vi "Start Module.vi"(8 "error in (no error)":errorcluster, 9 "Marca":T1, 10 "Com Port":refnum<visa-resource-name>, 11 "Run as Singleton? (F)":bool) -> (0 "error out":errorcluster, 1 "Wait for Event Sync?":bool, 2 "Multiple_uC Broadcast Events":T2, 3 "Module ID":i32)   [LabVIEW 2019, in "Multiple_uC.lvlib"]
doc: "Launches the Module Main.vi.\n_____\nBased on Delacor QMH Project Template 5.0.0.82."
uses:
  Multiple_uC.lvlib
  Broadcast Events--cluster.ctl
  Did Init Argument--cluster.ctl
  Status Updated Argument--cluster.ctl
  Error Reported Argument--cluster.ctl
  Stop Argument--cluster.ctl
  Get Module Execution Status Argument--cluster.ctl
  Clase Padre/Marca.ctl
  Module Running State--enum.ctl
  <vilib>/Delacor/Delacor QMH/Libraries/Cloneable Module Admin_class/Delacor_lib_QMH_Cloneable Module Admin.lvclass
  C:/Program Files/National Instruments/LabVIEW 2019/vi.lib/Delacor/Delacor QMH/Libraries/Module Admin_class/Delacor_lib_QMH_Module Admin.lvclass
  VI Reference Management/Main VI Type--strict_vi_ref.ctl
  <vilib>/Delacor/Delacor QMH/Libraries/Cloneable Module Admin_class/Delacor_lib_QMH_Cloneable Module Admin.lvclass/Delacor_lib_QMH_Cloneable Module Admin.ctl
  <vilib>/Delacor/Delacor QMH/Libraries/Module Admin_class/Delacor_lib_QMH_Module Admin.lvclass/Delacor_lib_QMH_Module Admin.ctl
  <vilib>/Delacor/Delacor QMH/Libraries/Cloneable Module Admin_class/Delacor_lib_QMH_Set Module ID.vi
  <vilib>/Delacor/Delacor QMH/Libraries/Module Admin_class/Delacor_lib_QMH_Set External Launch.vi
  <vilib>/Utility/error.llb/Error Cluster From Error Code.vi
  <vilib>/ErrorRing/Error Ring.xnode
  Clone Registration/Clone Registration.lvlib
  VI Reference Management/VI Reference Management.lvlib
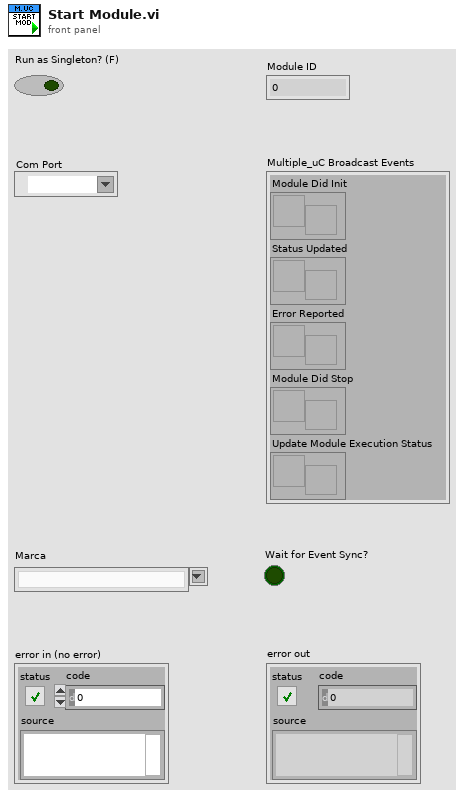
[diagram p1: front panel]
types:
  T1 = typedef "Marca.ctl" = string
  T2 = typedef "Multiple_uC.lvlib/Broadcast Events--cluster.ctl" = cluster{"Module Did Init":refnum<user-event>, "Status Updated":refnum<user-event>, "Error Reported":refnum<user-event>, "Module Did Stop":refnum<user-event>, "Update Module Execution Status":refnum<user-event>}
  T3 = typedef "Multiple_uC.lvlib/Module Running State--enum.ctl" = enum16{"Not Running", "Running as Cloneable", "Running as Singleton"}
  T4 = enum32{"Bad", "Idle", "Run top level", "Running"}
  T5 = typedef "Multiple_uC.lvlib/VI Reference Management.lvlib/Main VI Type--strict_vi_ref.ctl" = refnum<vi>
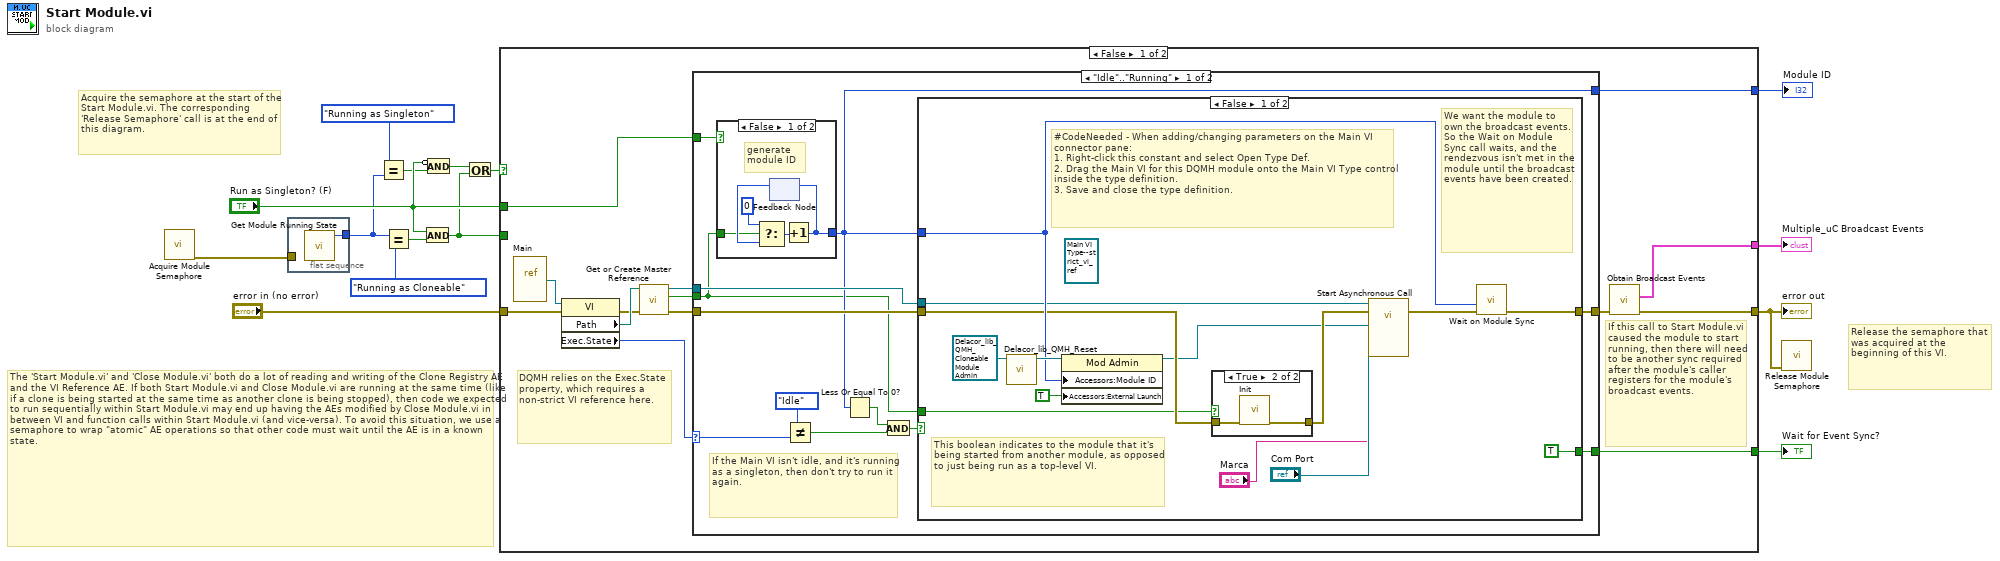
[diagram p0: block diagram]
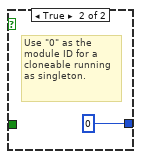
[diagram p2: hidden frame]
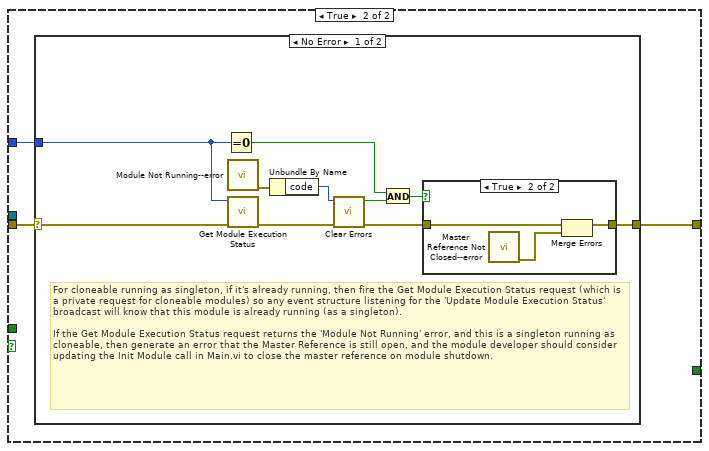
[diagram p4: hidden frame]
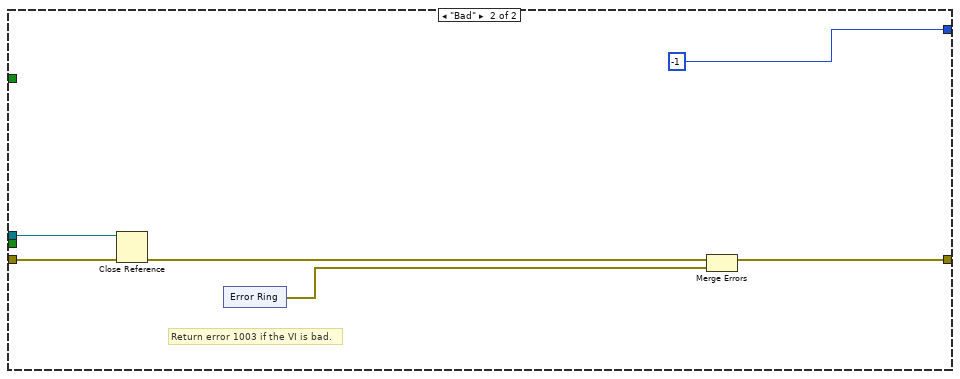
[diagram p7: hidden frame]
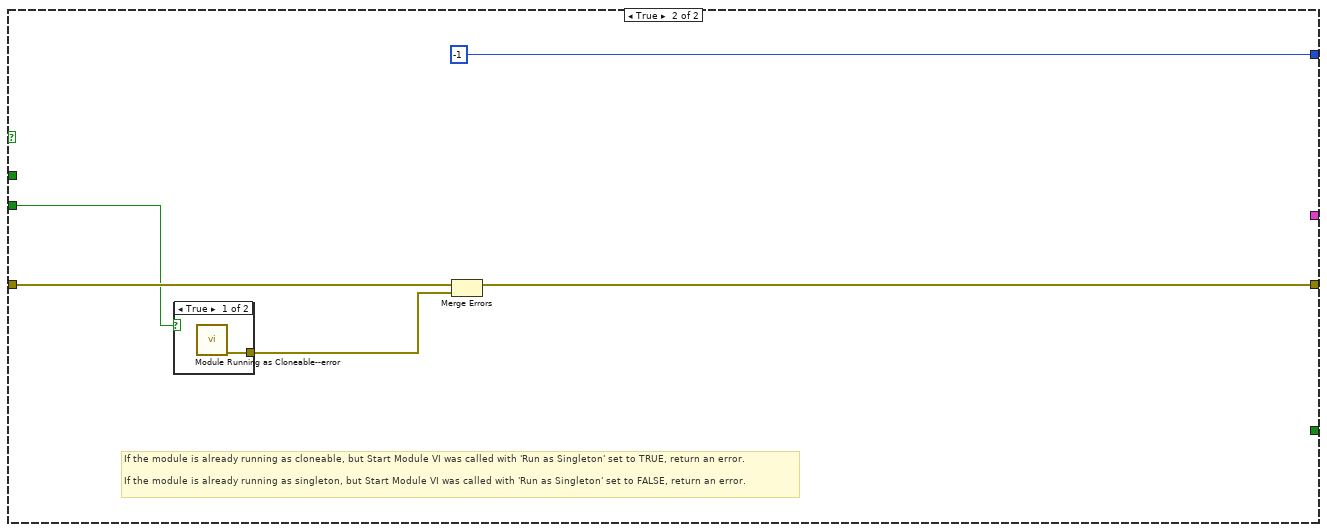
[diagram p8: hidden frame]
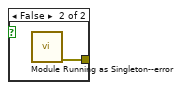
[diagram p9: hidden frame]
diagram:
  # "Release the semaphore that was acquired at the beginning of this VI."
  # "The 'Start Module.vi' and 'Close Module.vi' both do a lot of reading and writing of the Clone Registry AE and the VI Reference AE. If both Start Module.vi and Close Module.vi are running at the same time (like if a clone is being started at the same time as another clone is being stopped), then code we expected to run sequentially within Start Module.vi may end up having the AEs modified by Close Module.vi in between VI and function calls within Start Module.vi (and vice-versa). To avoid this situation, we use a semaphore to wrap \"atomic\" AE operations so that other code must wait until the AE is in a known state."
  # "Acquire the semaphore at the start of the Start Module.vi. The corresponding 'Release Semaphore' call is at the end of this diagram."
  n1 = call "Acquire Module Semaphore.vi"() -> ("error out"=w2:errorcluster)  [unwired: 11 in]
  n2 = flat-sequence {
    tunnel: [w16] -> w5
    tunnel: w2 -> [_]
    frame #0 {
      n3 = call "Get Module Running State.vi"() -> ("Module Running State"=w16:T3)  [unwired: 11 in]
    }
  }
  n4 = Equal?(x=Module_Running_State--enum."Running as Singleton", y=w5) -> (x = y?=w6:bool)
  n5 = Equal?(x=w5, y=Module_Running_State--enum."Running as Cloneable") -> (x = y?=w10:bool)
  n6 = And(x="Run as Singleton? (F)", y=w10) -> (x .and. y?=w3:bool)
  n7 = Compound Arithmetic op=AND(invert "Run as Singleton? (F)", w6) -> (w8:bool)
  n8 = Or(x=w8, y=w3) -> (x .or. y?=w9:bool)
  n9 = case shown="False" w9 {
    tunnel: "error in (no error)" -> [w30 w98]
    tunnel: [w28 w97] -> w1
    tunnel: [w27 _] -> w14
    tunnel: [w26 _] -> w13
    tunnel: [w22 -1] -> w12
    tunnel: "Run as Singleton? (F)" -> [w18 _]
    tunnel: w3 -> [_ w94]
    frame False {
      # "DQMH relies on the Exec.State property, which requires a non-strict VI reference here."
      # "If this call to Start Module.vi caused the module to start running, then there will need to be another sync required after the module's caller registers for the module's broadcast events."
      n10 = vi-ref "Main.vi"() -> (w21:refnum<vi>)
      n11 = property class="VI"(reference=w21, error in=w30) -> (error out=w24:errorcluster, "Path"=w25:path, "Exec.State"=w19:T4)  [unwired: 1 out]
      n12 = call "Get or Create Master Reference.vi"("error in (no error)"=w24, "Main VI Path"=w25) -> ("error out"=w23:errorcluster, "New Reference Created"=w17:bool, "Master Reference"=w20:T5)  [unwired: 7 in]
      n13 = case shown="\"Idle\"..\"Running\"" w19 {
        selector: w19 -> [w38 _]
        tunnel: w23 -> [w42 w89]
        tunnel: w20 -> [w40 w88]
        tunnel: [w39 w86] -> w29
        tunnel: [w41 _] -> w26
        tunnel: [w33 -1] -> w22
        tunnel: w18 -> [w32 _]
        tunnel: w17 -> [w31 _]
        frame "Idle".."Running" {
          # "If the Main VI isn't idle, and it's running as a singleton, then don't try to run it again."
          n14 = case shown="False" w32 {
            tunnel: [w47 0] -> w33
            tunnel: w31 -> [w43 _]
            frame False {
              # "generate module ID"
              n15 = feedback #1() -> (w45:i32)  [unwired: 1 in]
              n16 = Select(t=0, s=w43, f=w45) -> (s? t:f=w46:i32)
              n17 = Increment(x=w46) -> (x+1=w47:i32)
              n18 = feedback-in #1(w47) -> ()
            }
            frame True {
              # "Use \"0\" as the module ID for a cloneable running as singleton."
            }
          }
          n19 = Not Equal?(x=T4."Idle", y=w38) -> (x != y?=w36:bool)
          n20 = Less Or Equal To 0?(x=w33) -> (x <= 0?=w34:bool)
          n21 = And(x=w34, y=w36) -> (x .and. y?=w35:bool)
          n22 = case shown="False" w35 {
            tunnel: w42 -> [w54 w67]
            tunnel: [TRUE _] -> w41
            tunnel: w40 -> [w53 _]
            tunnel: [w57 w66] -> w39
            tunnel: w33 -> [w58 w68]
            tunnel: w31 -> [w51 _]
            frame False {
              (unwired) T5 refnum ("Main VI Type")
              # "#CodeNeeded - When adding/changing parameters on the Main VI connector pane:\n1. Right-click this constant and select Open Type Def.\n2. Drag the Main VI for this DQMH module onto the Main VI Type control inside the type definition.\n3. Save and close the type definition."
              # "We want the module to own the broadcast events. So the Wait on Module Sync call waits, and the rendezvous isn't met in the module until the broadcast events have been created."
              # "This boolean indicates to the module that it's being started from another module, as opposed to just being run as a top-level VI."
              n23 = call-dynamic "Delacor_lib_QMH_Reset.vi"("Mod Admin in"=refnum<class "Delacor_lib_QMH_Cloneable Module Admin.lvclass"> refnum) -> ("Mod Admin out"=w61:refnum<class "Delacor_lib_QMH_Cloneable Module Admin.lvclass">)  [unwired: 9 in, 1 out]
              n24 = property class="Mod Admin"(reference=w61, "Accessors:Module ID"=w58, "Accessors:External Launch"=TRUE) -> (reference out=w52:refnum<class "Delacor_lib_QMH_Cloneable Module Admin.lvclass">)  [unwired: 1 in, 1 out]
              n25 = case shown="True" w51 {
                tunnel: [w63 w65] -> w55
                tunnel: w54 -> [w63 w64]
                frame False {
                }
                frame True {
                  n26 = call "Init.vi"("error in (no error)"=w64) -> ("error out"=w65:errorcluster)  [unwired: 7 in, 3 out]
                }
              }
              n27 = call-by-ref "Start Asynchronous Call"(reference=w53, error in=w55, "Marca"="Marca", "Com Port"="Com Port", "Module Admin"=w52) -> (error out=w56:errorcluster)  [unwired: 9 in, 1 out]
              n28 = call "Wait on Module Sync.vi"("error in (no error)"=w56, "Module ID"=w58) -> ("error out"=w57:errorcluster)  [unwired: 9 in]
            }
            frame True {
              n29 = case shown="No Error" w67 {
                selector: w67 -> [w78 w83]
                tunnel: w68 -> [w76 _]
                tunnel: [w69 w83] -> w66
                frame No Error {
                  # "For cloneable running as singleton, if it's already running, then fire the Get Module Execution Status request (which is a private request for cloneable modules) so any event structure listening for the 'Update Module Execution Status' broadcast will know that this module is already running (as a singleton).\n\nIf the Get Module Execution Status request returns the 'Module Not Running' error, and this is a singleton running as cloneable, then generate an error that the Master Reference is still open, and the module developer should consider updating the Init Module call in Main.vi to close the master reference on module shutdown."
                  n30 = Equal To 0?(x=w76) -> (x = 0?=w72:bool)
                  n31 = call "Module Not Running--error.vi"() -> ("error out"=w75:errorcluster)  [unwired: 11 in]
                  n32 = call "Get Module Execution Status.vi"("error in (no error)"=w78, "Module ID"=w76) -> ("error out"=w77:errorcluster)  [unwired: 9 in]
                  n33 = Unbundle By Name(w75) -> ("code"=w74:i32)
                  n34 = call <vilib>:"Clear Errors.vi"("error in (no error)"=w77, "specific error code to clear (0: all)"=w74) -> ("error out"=w71:errorcluster, "specific error cleared?"=w73:bool)  [unwired: 4 in]
                  n35 = And(x=w72, y=w73) -> (x .and. y?=w70:bool)
                  n36 = case shown="True" w70 {
                    tunnel: w71 -> [w79 w82]
                    tunnel: [w79 w80] -> w69
                    frame False {
                    }
                    frame True {
                      n37 = call "Master Reference Not Closed--error.vi"() -> ("error out"=w81:errorcluster)  [unwired: 11 in]
                      n38 = Merge Errors(w82, w81) -> (w80:errorcluster)
                    }
                  }
                }
                frame Error {
                }
              }
            }
          }
        }
        frame "Bad" {
          # "Return error 1003 if the VI is bad."
          n39 = Close Reference(reference=w88, error in (no error)=w89) -> (error out=w87:errorcluster)
          n40 = xnode "Error Ring"() -> ("error out"=w85:errorcluster)
          n41 = Merge Errors(w87, w85) -> (w86:errorcluster)
        }
      }
      n42 = call "Obtain Broadcast Events.vi"("error in (no error)"=w29) -> ("error out"=w28:errorcluster, "Multiple_uC Broadcast Events"=w27:T2)  [unwired: 9 in]
    }
    frame True {
      # "If the module is already running as cloneable, but Start Module VI was called with 'Run as Singleton' set to TRUE, return an error.\n\nIf the module is already running as singleton, but Start Module VI was called with 'Run as Singleton' set to FALSE, return an error."
      n43 = case shown="True" w94 {
        tunnel: [w99 w100] -> w95
        frame True {
          n44 = call "Module Running as Cloneable--error.vi"() -> ("error out"=w99:errorcluster)  [unwired: 11 in]
        }
        frame False {
          n45 = call "Module Running as Singleton--error.vi"() -> ("error out"=w100:errorcluster)  [unwired: 11 in]
        }
      }
      n46 = Merge Errors(w98, w95) -> (w97:errorcluster)
    }
  }
  "error out" <- w1
  "Multiple_uC Broadcast Events" <- w14
  "Wait for Event Sync?" <- w13
  "Module ID" <- w12
  n47 = call "Release Module Semaphore.vi"("error in"=w1) -> ()  [unwired: 10 in, 1 out]
